vi "add_to_arrays.vi"(8 "index":i32, 9 "min dip":dbl, 10 "steepest slope":dbl, 11 "initialized arrays":cluster{dbl[], dbl[]}) -> (3 "arrays out":cluster{dbl[], dbl[]})   [LabVIEW 2015]
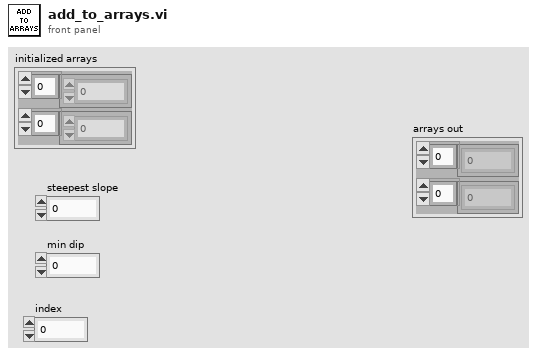
[diagram p1: front panel]
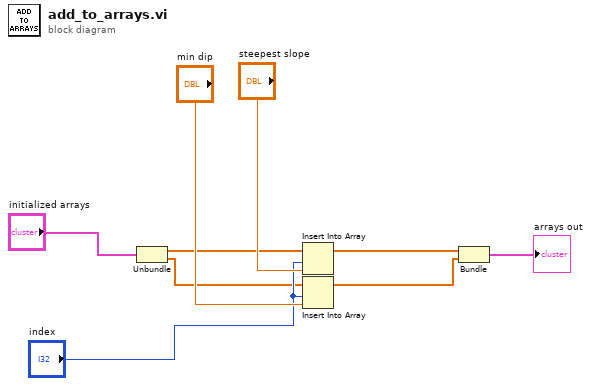
[diagram p0: block diagram]
diagram:
  n1 = Unbundle("initialized arrays") -> (w5:dbl[], w4:dbl[])
  n2 = Insert Into Array(array=w5, index="index", new element="steepest slope") -> (w3:dbl[])
  n3 = Insert Into Array(array=w4, index="index", new element="min dip") -> (w2:dbl[])
  n4 = Bundle(w3, w2) -> (→"arrays out":cluster{dbl[], dbl[]})  [unwired: 1 in]
